vi "DeInit.vi"(8 "error in (no error)":errorcluster, 11 "HRS_Spectrometer in":refnum<class "HRS_Spectrometer.lvclass">) -> (0 "error out":errorcluster, 3 "HRS_Spectrometer out":refnum<class "HRS_Spectrometer.lvclass">)   [LabVIEW 2023, in "HRS_Spectrometer.lvlib" / "HRS_Spectrometer.lvclass"]
uses:
  HRS_Spectrometer.lvclass
  HRS_Spectrometer.lvclass/HRS_Spectrometer.ctl
  <vilib>/Instr/_visa.llb/Select Event Type.ctl
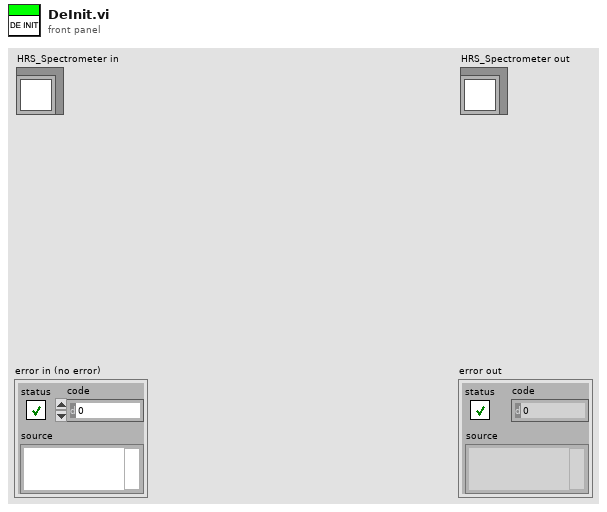
[diagram p1: front panel]
types:
  T1 = typedef "Select Event Type.ctl" = u32
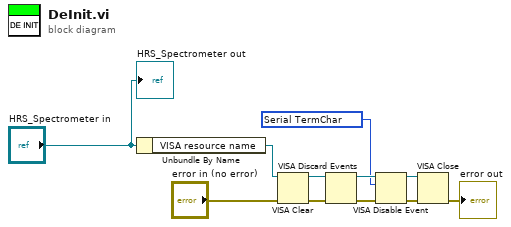
[diagram p0: block diagram]
diagram:
  w1 = T1 1073684516 items=["Service Request"=1073684491, "Trigger"=3221168138, "Clear"=1073684493, "VXI Signal"=1073684512, "VXI/VME Interrupt"=3221168161, "VXI/VME Sysfail"=1073684509, "VXI/VME Sysreset"=1073684510, "GPIB CIC"=1073684498, "GPIB Talk"=1073684499, "GPIB Listen"=1073684500, "PXI Interrupt"=1073684514, "Serial Break"=1073684515, "Serial TermChar"=1073684516, "Serial CTS"=1073684521, "Serial DSR"=1073684522, "Serial DCD"=1073684524, "Serial RI"=1073684526, "Serial Character"=1073684533, "USB Interrupt"=1073684535, "All Enabled"=1073709055] ("Event Type")
  n1 = Unbundle By Name("HRS_Spectrometer in") -> ("VISA resource name"=w10:refnum<visa-resource-name>)
  n2 = VISA Clear(VISA resource name=w10, error in (no error)="error in (no error)") -> (VISA resource name out=w5:refnum<visa-resource-name>, error out=w3:errorcluster)
  n3 = VISA Discard Events(8:w3, 11:w5) -> (0:w6:errorcluster, 3:w7:refnum<visa-resource-name>)  [unwired: 2 in]
  n4 = VISA Disable Event(8:w6, 10:w1, 11:w7) -> (0:w2:errorcluster, 3:w4:refnum<visa-resource-name>)  [unwired: 1 in]
  n5 = VISA Close(VISA resource name=w4, error in (no error)=w2) -> (error out=→"error out":errorcluster)
  "HRS_Spectrometer out" <- "HRS_Spectrometer in"
